vi "EnviraCom_ON_OFF.vi"(8 "error in (no error)":errorcluster, 10 "ON (True), OFF (False)":bool, 11 "VISA Refnum in":refnum<visa-resource-name>) -> (0 "error out":errorcluster, 3 "VISA Refnum out":refnum<visa-resource-name>)   [LabVIEW 2023]
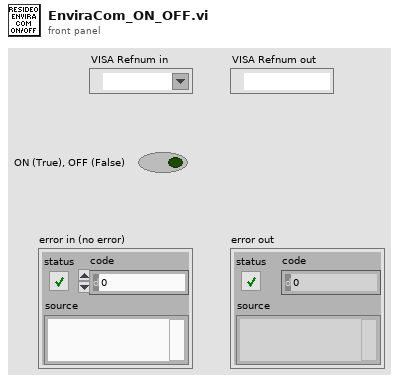
[diagram p1: front panel]
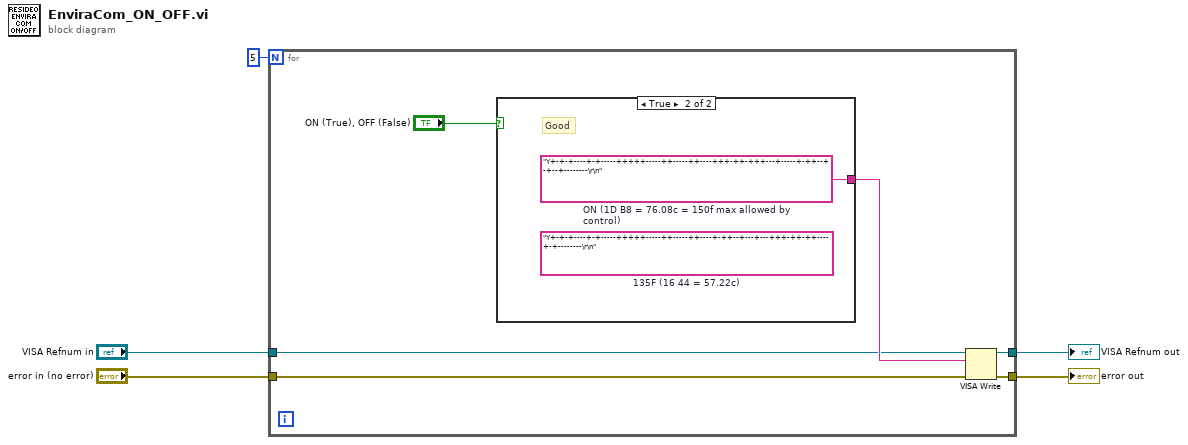
[diagram p0: block diagram]
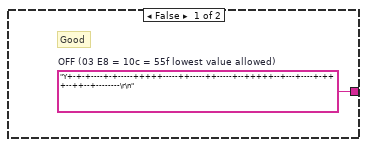
[diagram p2: hidden frame]
diagram:
  n1 = for {
    N: 5 -> [_]
    tunnel: "VISA Refnum in" -> [w8]
    tunnel: [w9] -> w5
    tunnel: "error in (no error)" -> [w6]
    tunnel: [w7] -> w3
    n2 = case shown="True" "ON (True), OFF (False)" {
      tunnel: [w12 w13] -> w10
      frame False {
        w12 = "Y+-+-+----+-+-----+++++-----++-----++-----+--+++++--+---+----+-+++--++--+--------\r\n"  # OFF (03 E8 = 10c = 55f lowest value allowed)
        # "Good"
      }
      frame True {
        (unwired) "Y+-+-+----+-+-----+++++-----++-----++----+-++--+---+---+++-++-++----+-+--------\r\n"  # 135F (16 44 = 57.22c)
        w13 = "Y+-+-+----+-+-----+++++-----++-----++----+++-++-+++---+-----+-++--+-+--+--------\r\n"  # ON (1D B8 = 76.08c = 150f max allowed by control)
        # "Good"
      }
    }
    n3 = VISA Write(VISA resource name=w8, write buffer=w10, error in (no error)=w6) -> (VISA resource name out=w9:refnum<visa-resource-name>, error out=w7:errorcluster)  [unwired: 1 out]
  }
  "VISA Refnum out" <- w5
  "error out" <- w3
